vi "PickAndDestroy.vi"(0 "ImageIn":T1, 4 "Threshold":dbl=20.0 format="%.2f", 5 "Image":u32[][](array[numeric]), 6 "Image Settings":T4 {"2nd Axis" items=["x", "y", "z"]; "1st Axis" items=["x", "y", "z"]; "Time Resolution\n(ms/pixel)" format="%.2f"; "Image Resolution (nm/pixel)"."z" format="%.2f"; "Image Resolution (nm/pixel)"."y" format="%.2f"; "Image Resolution (nm/pixel)"."x" format="%.2f"; "Image Size (µm)"."z" format="%.2f"; "Image Size (µm)"."y" format="%.2f"; "Image Size (µm)"."x" format="%.2f"; "End Position (µm)"."z" format="%.2f"; "End Position (µm)"."y" format="%.2f"; "End Position (µm)"."x" format="%.2f"; "Start Position (µm)"."z" format="%.2f"; "Start Position (µm)"."y" format="%.2f"; "Start Position (µm)"."x" format="%.2f"}) -> ()   [LabVIEW 2009]
uses:
  ImageSettings.ctt
  <vilib>/vision/Image Controls.llb/IMAQ Image.ctl
  AO Update Channel (scaled value).vi
  <vilib>/ptbypt/NI_PtbyPt.lvlib
panel:
  out "spots left":i32
  out "Boolean":bool
  out "sum":i32
  in  "AutoFocus Z":bool
  in  "Delay Time (s)":dbl=120.0
  out "autofocus stub":i32[](array[numeric])
  out "Debug Image Ints":T1(plugin-control)
  out "Intensity for ft debug color/rotated by some angle":dbl[][](graph)
  out "Intensity fit gausian for SM":dbl[][](graph)
  in  "radius":i32
  out "Focuswidth/px":dbl
  in  "Treshold":dbl
  out "NrOfSpots":i32
  in  "Find Molecules":bool
  in  "Automate Mesaurement":bool
  in  "Focuswidth nm":dbl
  in  "AFM mode":bool
  in  "gauss fit":bool
  in  "channel":i32
  in  "initialize":bool
  out "Histogram Graph":T2(graph)
  in  ".sm file format":bool
  in  "manual positioning":cluster{"x":dbl, "y":dbl, "z":dbl}
  in  "Laser 4":bool
  out "used":bool
  in  "Ramp Setup":bool
  in  "% duration Laser1":u8=50 min=1 max=99
  in  "% puls-duration":dbl=100.0
  in  "Laser 3":bool
  in  "Laser 2":bool
  in  "Laser 1":bool
  in  "AOTF Setup":bool
  in  "AOTF":u16(ring)=1 items=["None", "Laser 1", "Laser 2", "Laser 1 + 2", "Laser 3", "Laser 1 + 3", "Laser 2 + 3", "Laser 1+2+3", "Laser 1+2+3+4", "Laser 2+3+4"]
  out "Pickcoord. (pixel)":cluster{dbl, dbl, dbl}
  in  "offset (pixel)":cluster{dbl, dbl, dbl}
  out "coordinates (pixel)":cluster{dbl, dbl, dbl}
  out "Actual Spot No.":u32
  in  "Store Pick Image":bool
  in  "Next":bool caption="Run"
  in  "Show MCS":bool=TRUE
  in  "Pick Settings":T3={"Automatic"=FALSE, "Threshold"=20.0, "radius"=0} {"Threshold" format="%.2f"}
  in  "Run":bool
  in  "Destination:":path
  in  "Store Data":bool caption="Store Data:"
  in  "Stage Setup":bool
  in  "SPC Setup":bool
  in  "EOM Setup":bool
  in  "EOM":u16(ring) items=["None", "Trace", "Retrace", "All"]
  out "Counts":cluster{"Total":u32, "Gap":u32, "Invalid":u32}
  out "MCS":i32[][](graph)
  in  "Exit":bool
  # "+"
  # "="
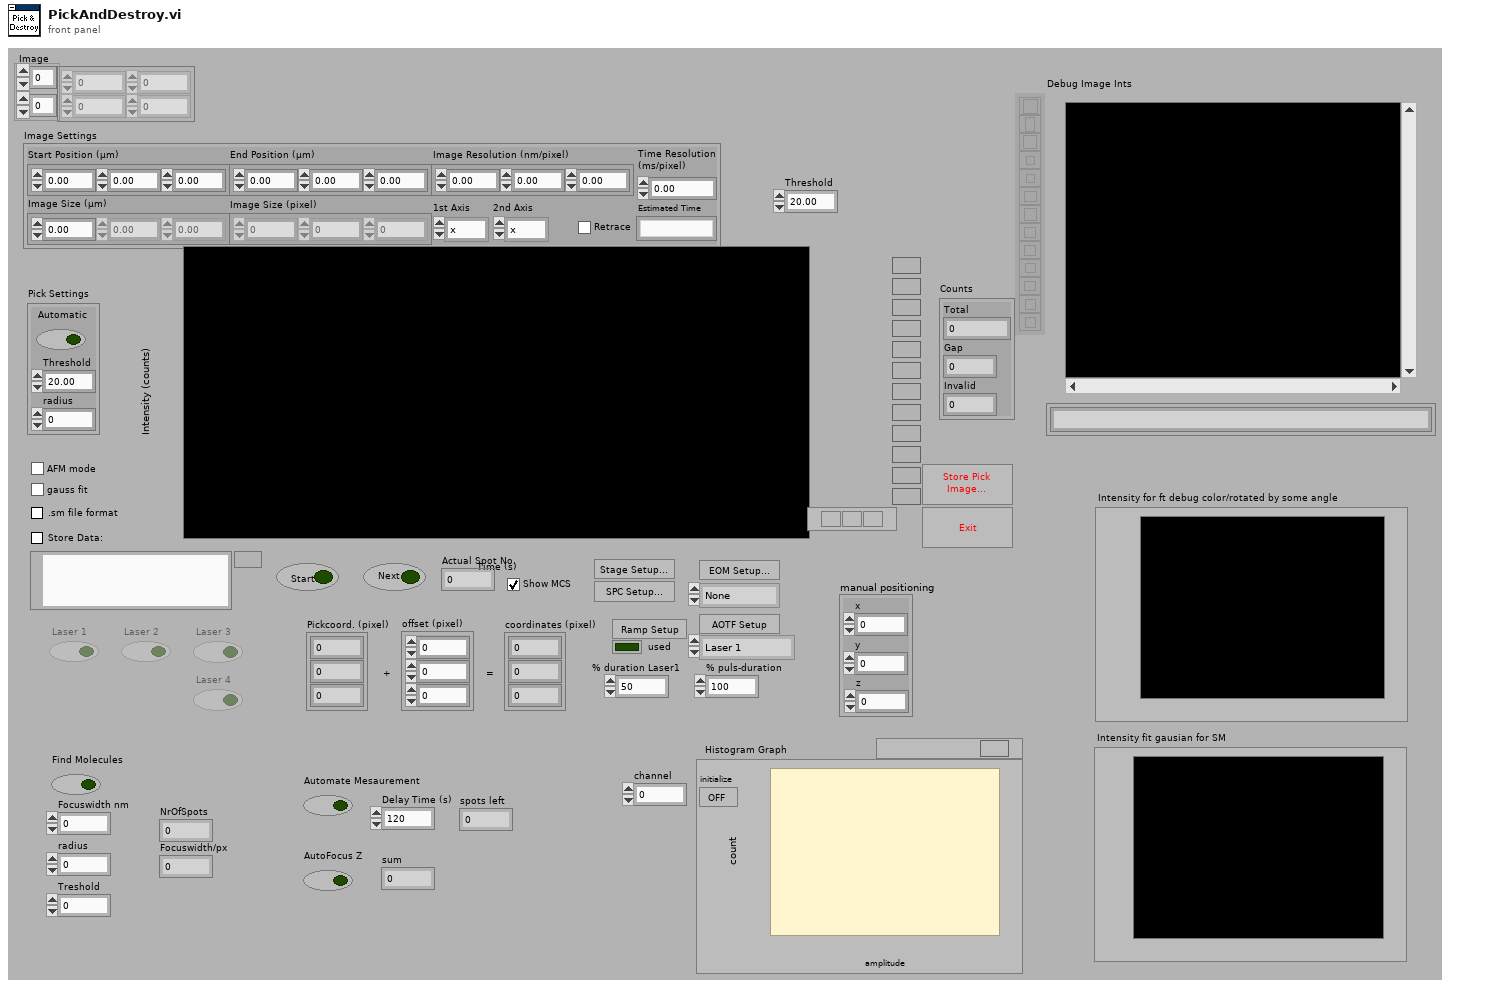
[diagram p1: front panel]
types:
  T1 = typedef "IMAQ Image.ctl" = refnum<image>
  T2 = cluster{"X Values":dbl[], "Histogram: h(x)":i32[]}
  T3 = cluster{"Automatic":bool, "Threshold":dbl, "radius":i32}
  T4 = typedef "ImageSettings.ctt" = cluster{"Start Position (µm)":cluster{"x":dbl, "y":dbl, "z":dbl}, "End Position (µm)":cluster{"x":dbl, "y":dbl, "z":dbl}, "Image Resolution (nm/pixel)":cluster{"x":dbl, "y":dbl, "z":dbl}, "Image Size (µm)":cluster{"x":dbl, "y":dbl, "z":dbl}, "Image Size (pixel)":cluster{"x":u32, "y":u32, "z":u32}, "Time Resolution\n(ms/pixel)":dbl, "1st Axis":u16, "2nd Axis":u16, "Retrace":bool, "Estimated Time":string}
  T5 = enum16{"Get Type", "Set Type", "GetStageInit", "GetWriteStageSetting", "GetInitializeStageOutput", "GetSetAxisPosition", "GetSetPos", "GetSetupStage", "HaltStageOutput"}
  T6 = typedef "FIFOSettings.ctt" = cluster{"Measurement":cluster{"Binning (ms)":sgl, "External Trigger Condition":u16, "Stop Condition:":u16, "Stop Count":dbl, "Buffer Size (Photons)":u32, "No of Channels":u16, "Ext Latch Delay":i16}, "ADC":cluster{"Binning (HH)":i16, "Dither Range":i16, "Count Increment":i16, "Mode":u16}, "SYNC":cluster{"SYNC ZC Level (mV)":sgl, "SYNC Freq Divider":u16, "SYNC Holdoff (ps)":sgl, "SYNC Threshold (mV)":sgl}, "TAC":cluster{"TAC Range (ns)":sgl, "TAC Gain":i16, "TAC Offset (%)":sgl, "TAC Limit Low (%)":sgl, "TAC Limit High (%)":sgl}, "Ch 2":cluster{"Ch2 ZC Level (mV)":sgl, "Ch2 Holdoff (ps)":sgl, "Ch2 Threshold (mV)":sgl}, "Ch 3":cluster{"Ch3 ZC Level (mV)":sgl, "Ch3 Holdoff (ps)":sgl, "Ch3 Threshold (mV)":sgl}, "Ch 4":cluster{"Ch4 ZC Level (mV)":sgl, "Ch4 Holdoff (ps)":sgl, "Ch4 Threshold (mV)":sgl}, "Ch1":cluster{"Ch1 ZC Level (mV)":sgl, "Ch1 Holdoff (ps)":sgl, "Ch1 Threshold (mV)":sgl}}
  T7 = typedef "PickImage.ctl" = cluster{"Rawdata":T1, "Mask":T1, "Display":T1, "Coefficients (2D)":sgl[][], "Destroy Index":u32}
  T8 = cluster{"Binning (ms)":sgl, "External Trigger Condition":u16, "Stop Condition:":u16, "Stop Count":dbl, "Buffer Size (Photons)":u32, "No of Channels":u16, "Ext Latch Delay":i16}
  T9 = cluster{"router channels":u8[], "macro times(50ns steps)":u32[], "micro times":u16[], "invalid times":u32[], "gap times":u32[]}
  T10 = cluster{"Start Position (µm)":cluster{"x":dbl, "y":dbl, "z":dbl}, "End Position (µm)":cluster{"x":dbl, "y":dbl, "z":dbl}, "Image Resolution (nm/pixel)":cluster{"x":dbl, "y":dbl, "z":dbl}, "Image Size (µm)":cluster{"x":dbl, "y":dbl, "z":dbl}, "Image Size (pixel)":cluster{"x":u32, "y":u32, "z":u32}, "Time Resolution\n(ms/pixel)":dbl, "1st Axis":u16, "2nd Axis":u16, "Retrace":bool, "Estimated Time":string}
  T11 = typedef "StageType.ctt" = enum16{"PI 725 USB", "PI 725 TCP/IP", "PI analogue step"}
  T12 = cluster{"used":bool, "steps":u16, "start (V)":dbl, "stop (V)":dbl, "periode (s)":dbl, "manual":dbl[][]}
  T13 = typedef "DAQLinescanVisualization.ctt" = cluster{"Threshold":u32, "Trace Window #":u32, "IMAQ Trace":T1, "Retrace Window #":u32, "IMAQ Retrace":T1}
  T14 = typedef "AOTFSettings.ctt" = cluster{"Laser 1 Output Channel":tag, "AOTF  1 Output Voltage":dbl, "Laser 2 Output Channel":tag, "AOTF  2 Output Voltage":dbl, "Laser 3 Output Channel":tag, "AOTF  3 Output Voltage":dbl, "Pixel per Cycle":u16, "Time per Cycle  / ms":dbl, "Laser 4 Output Channel":tag, "AOTF  4 Output Voltage":dbl, "Laser 5 Output Channel":tag, "AOTF 5 Output Voltage ":dbl, "Laser 6 Output Channel":tag, "AOTF  6 Output Voltage ":dbl, "Laser 7 Output Channel":tag, "AOTF 7 Output Voltage ":dbl, "Laser 8 Output Channel":tag, "AOTF  8 Output Voltage ":dbl, "AOTF  1 Frequency":dbl, "AOTF  2 Frequency":dbl, "AOTF  3  Frequency":dbl, "AOTF  4 Frequency":dbl, "AOTF 5 Frequency":dbl, "AOTF  6 Frequency":dbl, "AOTF 7  Frequency":dbl, "AOTF  8 Frequency":dbl, "AOTF  1 Amplitude":dbl, "AOTF  2 Amplitude":dbl, "AOTF  3  Amplitude":dbl, "AOTF  4 Amplitude":dbl, "AOTF 5 Amplitude":dbl, "AOTF  6 Amplitude":dbl, "AOTF 7 Amplitude  ":dbl, "AOTF  8 Amplitude":dbl}
  T15 = typedef "AnalogSettings.ctt" = cluster{"PCI 671x Device Number":u32, "Samples per Unit":u32}
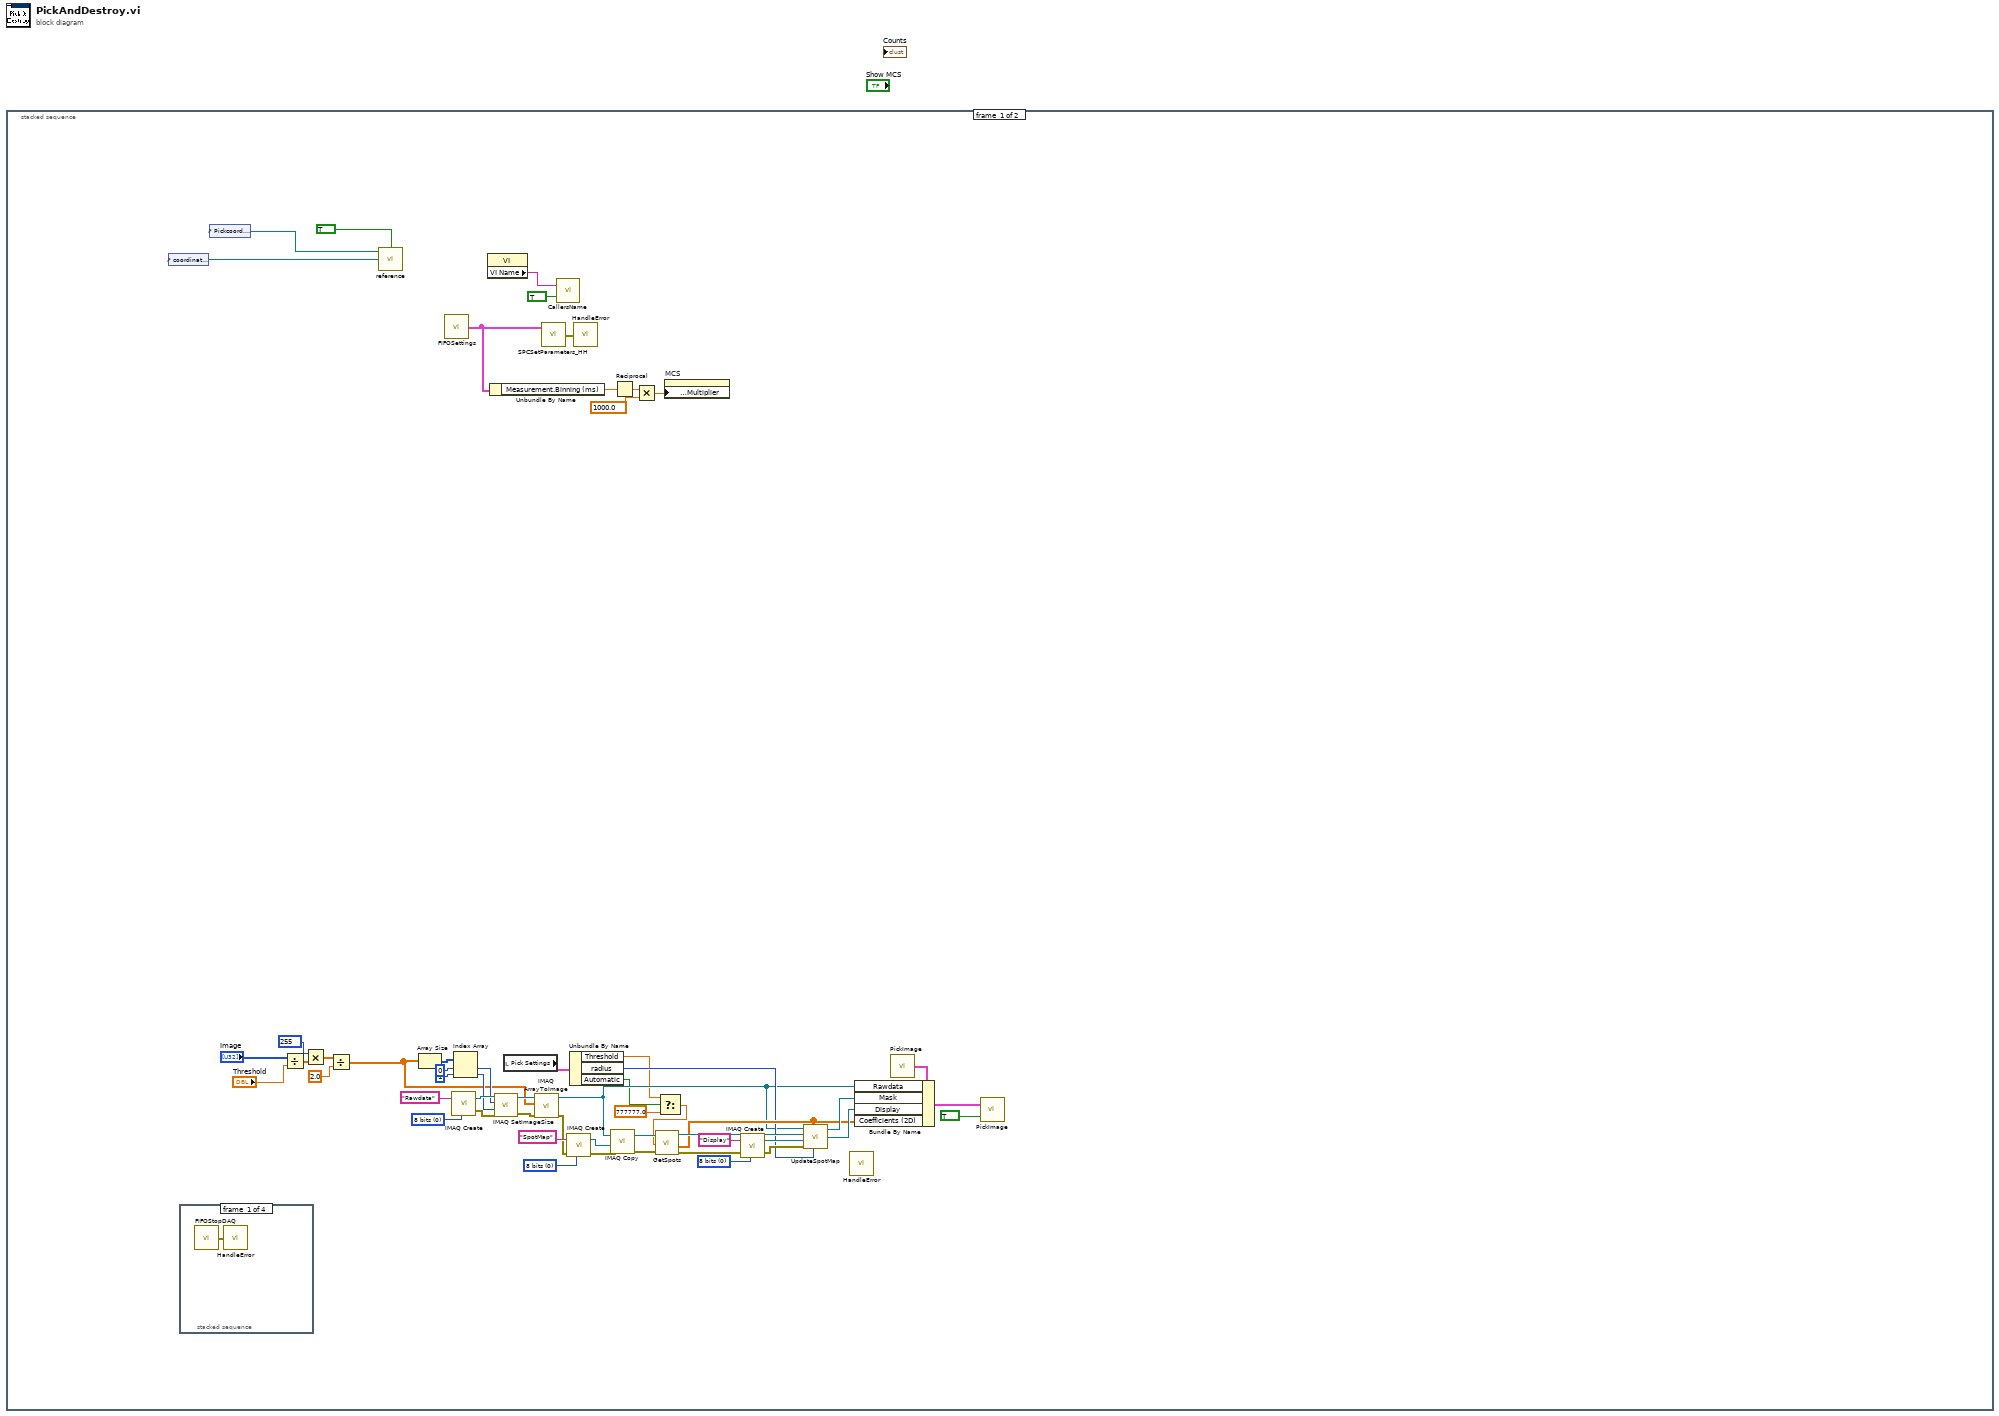
[diagram p0: block diagram]
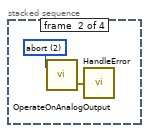
[diagram p2: hidden frame]
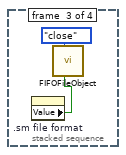
[diagram p3: hidden frame]
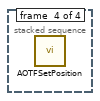
[diagram p4: hidden frame]
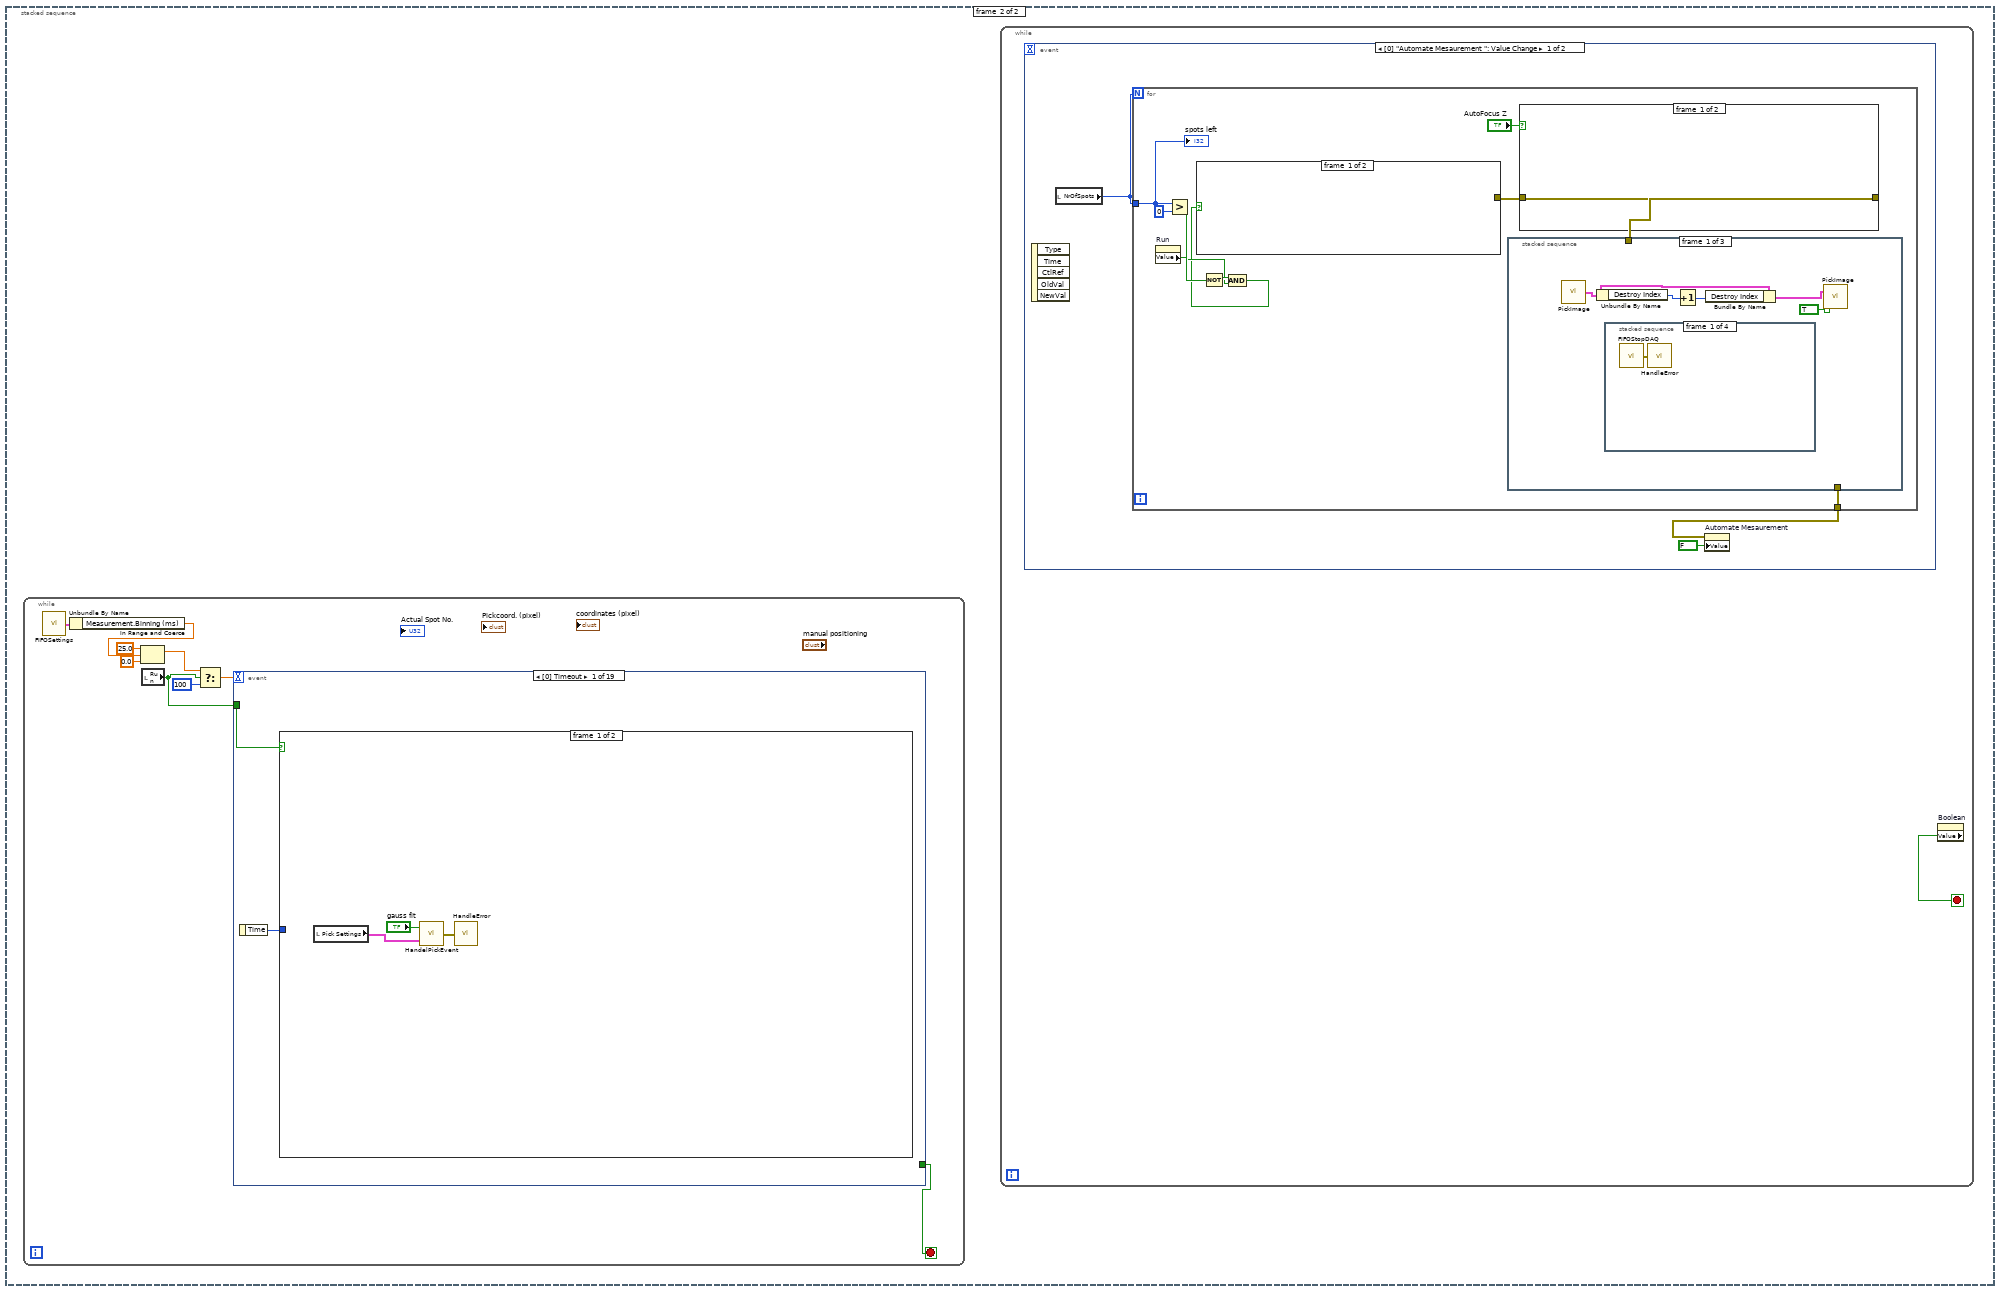
[diagram p5: hidden frame]
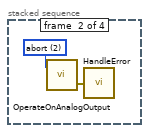
[diagram p6: hidden frame]
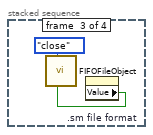
[diagram p7: hidden frame]
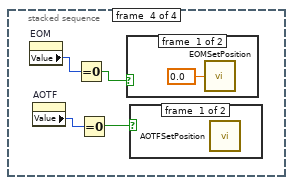
[diagram p8: hidden frame]
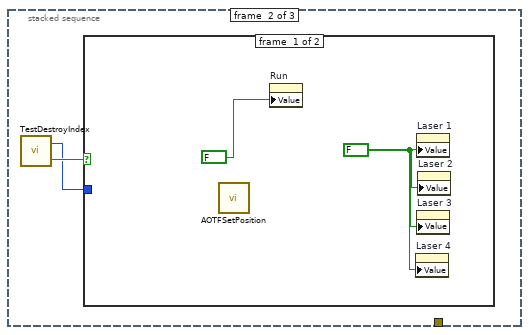
[diagram p11: hidden frame]
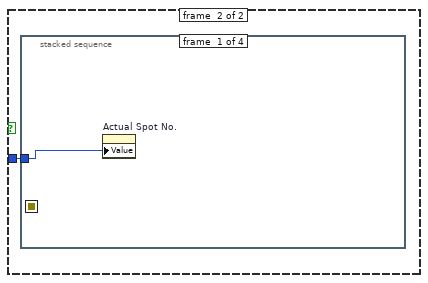
[diagram p12: hidden frame]
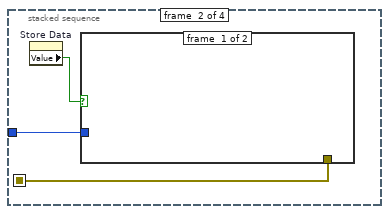
[diagram p13: hidden frame]
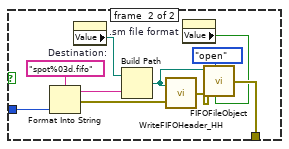
[diagram p14: hidden frame]
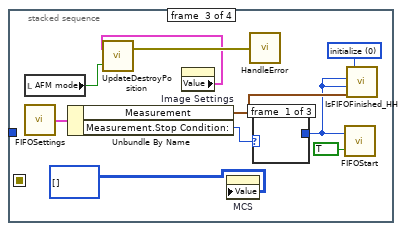
[diagram p15: hidden frame]
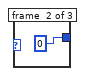
[diagram p16: hidden frame]
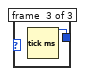
[diagram p17: hidden frame]
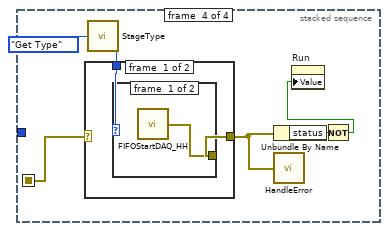
[diagram p18: hidden frame]
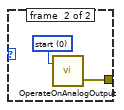
[diagram p19: hidden frame]
diagram:
  n1 = stacked-sequence {
    frame #0 {
      w39 = u32 0 items=["8 bits", "16 bits", "Float", "Complex", "RGB", "HSL"] ("Image Type")
      w44 = u32 0 items=["8 bits", "16 bits", "Float", "Complex", "RGB", "HSL"] ("Image Type")
      w54 = u32 0 items=["8 bits", "16 bits", "Float", "Complex", "RGB", "HSL"] ("Image Type")
      n2 = control-ref of="coordinates (pixel)"() -> (w16:refnum<vi>)
      n3 = stacked-sequence {
        frame #0 {
          n4 = call "FIFOStopDAQ.vi"() -> ("error out"=w56:errorcluster)
          n5 = call "HandleError.vi"("error in (no error)"=w56) -> ()
        }
        frame #1 {
          w58 = u16 2 items=["start", "state", "abort"] ("operation")
          n6 = call "OperateOnAnalogOutput.vi"("operation"=w58) -> ("error out"=w57:errorcluster)  [unwired: 1 in, 1 out]
          n7 = call "HandleError.vi"("error in (no error)"=w57) -> ()
        }
        frame #2 {
          n8 = property on=".sm file format" class="Bool (strict)"() -> ("Value"=w59:bool)  [unwired: 2 in, 2 out]
          n9 = call "FIFOFileObject.vi"(".sm file format"=w59, "function (open:0)"=enum16{"open", "write", "close"}."close") -> ()  [unwired: 4 in, 1 out]
        }
        frame #3 {
          n10 = call "AOTFSetPosition.vi"() -> ()  [unwired: 2 in]
        }
      }
      n11 = control-ref of="Pickcoord. (pixel)"() -> (w17:refnum<vi>)
      n12 = Divide(x="Image", y="Threshold") -> (x/y=w22:dbl[][])
      n13 = Multiply(x=u8 255, y=w22) -> (x*y=w7:dbl[][])
      n14 = Divide(x=w7, y=2.0) -> (x/y=w5:dbl[][])
      n15 = call "reference.vi"("set?"=TRUE, "coordinates (pixel)"=w16, "Pickcoord. (pixel)"=w17) -> ()  [unwired: 1 in, 2 out]
      n16 = Array Size(array=w5) -> (size(s)=w53:i32[])
      n17 = call "FIFOSettings.vi"() -> ("FIFO Settings(out)"=w14:T6)  [unwired: 2 in]
      n18 = call "IMAQ Create"("Image Name"="Rawdata", "Image Type"=w54) -> ("New Image"=w50:T1, "error out"=w49:errorcluster)  [unwired: 3 in]
      n19 = Index Array(array=w53, index #1=0 ("index"), index #2=1 ("index")) -> (element #1=w8:i32, element #2=w38:i32)
      n20 = property class="VI"() -> ("VI Name"=w18:string)  [unwired: 2 in, 2 out]
      n21 = Unbundle By Name(w14) -> ("Measurement.Binning (ms)"=w13:sgl)
      n22 = call "IMAQ SetImageSize"("error in (no error)"=w49, "Y Resolution"=w38, "X Resolution"=w8, "Image"=w50) -> ("error out"=w47:errorcluster, "Image Out"=w48:T1)  [unwired: 1 in]
      n23 = local read "Pick Settings"() -> (w26:T3)
      n24 = call "IMAQ ArrayToImage"("error in (no error)"=w47, "Image Pixels (U8)"=w5, "Image"=w48) -> ("error out"=w41:errorcluster, "Image Out"=w9:T1)  [unwired: 7 in]
      n25 = call "SPCSetParameters_HH.vi"("FIFO Settings"=w14) -> ("error (out)"=w24:errorcluster)  [unwired: 2 in]
      n26 = call "CallersName.vi"("Get/Set"=TRUE ("s"), "Callers Name"=w18) -> ()  [unwired: 1 out]
      n27 = call "IMAQ Create"("Image Name"="SpotMap", "Image Type"=w44, "error in (no error)"=w41) -> ("New Image"=w37:T1, "error out"=w36:errorcluster)  [unwired: 2 in]
      n28 = Unbundle By Name(w26) -> ("Threshold"=w4:dbl, "radius"=w25:i32, "Automatic"=w3:bool)
      n29 = call "HandleError.vi"("error in (no error)"=w24) -> ()
      n30 = call "IMAQ Copy"("error in (no error)"=w36, "Image Dst"=w37, "Image Src"=w9) -> ("error out"=w34:errorcluster, "Image Dst Out"=w35:T1)  [unwired: 3 in]
      n31 = Reciprocal(x=w13) -> (1/x=w12:sgl)
      n32 = Multiply(x=w12, y=sgl 1000.0) -> (x*y=w11:sgl)
      n33 = Select(t=w4, s=w3, f=777777.0) -> (s? t:f=w1:dbl)
      n34 = call "GetSpots.vi"("New Image"=w35, "Threshold"=w1, "error in (no error)"=w34) -> ("Image Dst Out"=w30:T1, "Coefficients (2D)"=w27:sgl[][], "error out"=w33:errorcluster)  [unwired: 2 out]
      n35 = property on="MCS" class="WFChart (strict)"("X Scale.Offset and Multiplier:Multiplier"=w11) -> ()  [unwired: 2 in, 2 out]
      n36 = call "IMAQ Create"("Image Name"="Display", "Image Type"=w39, "error in (no error)"=w33) -> ("New Image"=w31:T1, "error out"=w32:errorcluster)  [unwired: 2 in]
      n37 = call "UpdateSpotMap.vi"("Rawdata"=w9, "Coefficients"=w27, "Mask (input)"=w30, "Display Input"=w31, "radius"=w25, "error in (no error)"=w32) -> ("Mask (output)"=w29:T1, "Display (output"=w28:T1)  [unwired: 1 out]
      n38 = call "HandleError.vi"() -> ()  [unwired: 1 in]
      n39 = call "PickImage.vi"() -> ("Image (output)"=w46:T7)  [unwired: 2 in]
      n40 = Bundle By Name(cluster=w46, "Rawdata"=w9, "Mask"=w29, "Display"=w28, "Coefficients (2D)"=w27) -> (w42:T7)
      n41 = call "PickImage.vi"("Get/Set"=TRUE, "Images (input)"=w42) -> ()  [unwired: 1 out]
    }
    frame #1 {
      n42 = while {
        stop <- w154 stop-if-true
        n43 = call "FIFOSettings.vi"() -> ("FIFO Settings(out)"=w150:T6)  [unwired: 2 in]
        n44 = Unbundle By Name(w150) -> ("Measurement.Binning (ms)"=w147:sgl)
        n45 = In Range and Coerce(upper limit=25.0, x=w147, lower limit=0.0) -> (coerced(x)=w146:dbl)  [unwired: 1 out]
        n46 = local read "Run"() -> (w151:bool)
        n47 = Select(t=w146, s=w151, f=100) -> (s? t:f=w152:dbl)
        n48 = event shown="[0] Timeout" {
          selector: _ -> [_ _ _ _ _ _ _ _ _ _ _ _ _ _ _ _ _ _ _]
          dyn-events: _ -> [_ _ _ _ _ _ _ _ _ _ _ _ _ _ _ _ _ _ _]
          timeout: w152 -> [_ _ _ _ _ _ _ _ _ _ _ _ _ _ _ _ _ _ _]
          tunnel: [_ _ _ _ _ _ _ _ _ _ _ _ _ _ _ _ _ _ w534] -> w154
          tunnel: w151 -> [w156 _ _ _ _ _ _ _ _ _ _ _ _ _ _ _ _ _ _]
          event #0 {
            n49 = event-data() -> ("Time"=w155:u32)  [unwired: 1 in]
            n50 = case shown="True" w156 {
              tunnel: w155 -> [_ w160]
              frame #0 {
                n51 = local read "Pick Settings"() -> (w159:T3)
                n52 = call "HandelPickEvent.vi"("Pick Settings"=w159, "gauss fit"="gauss fit") -> ("error out"=w158:errorcluster)
                n53 = call "HandleError.vi"("error in (no error)"=w158) -> ()
              }
              frame #1 {
                n54 = call "IsSPCArmed_HH.vi"() -> ("Boolean"=w161:bool)  [unwired: 1 in]
                n55 = case shown="True" w161 {
                  tunnel: w160 -> [w164 w206]
                  frame #0 {
                    n56 = call "TestDestroyIndex.vi"() -> ("Boolean"=w163:bool, "Destroy Index"=w162:u32)
                    n57 = case shown="True" w163 {
                      selector: w163 -> [w165 _]
                      tunnel: w164 -> [_ _]
                      tunnel: w162 -> [_ w171]
                      frame #0 {
                        n58 = property on="Run" class="Boolean (strict)"("Value"=w165) -> ()  [unwired: 2 in, 2 out]
                        n59 = stacked-sequence {
                          frame #0 {
                            n60 = call "FIFOStopDAQ.vi"() -> ("error out"=w166:errorcluster)
                            n61 = call "HandleError.vi"("error in (no error)"=w166) -> ()
                          }
                          frame #1 {
                            w168 = u16 2 items=["start", "state", "abort"] ("operation")
                            n62 = call "OperateOnAnalogOutput.vi"("operation"=w168) -> ("error out"=w167:errorcluster)  [unwired: 1 in, 1 out]
                            n63 = call "HandleError.vi"("error in (no error)"=w167) -> ()
                          }
                          frame #2 {
                            n64 = property on=".sm file format" class="Bool (strict)"() -> ("Value"=w169:bool)  [unwired: 2 in, 2 out]
                            n65 = call "FIFOFileObject.vi"(".sm file format"=w169, "function (open:0)"=enum16{"open", "write", "close"}."close") -> ()  [unwired: 4 in, 1 out]
                          }
                          frame #3 {
                            n66 = call "AOTFSetPosition.vi"() -> ()  [unwired: 2 in]
                            n67 = call "EOMSetPosition.vi"() -> ()  [unwired: 1 in]
                          }
                        }
                      }
                      frame #1 {
                        n68 = stacked-sequence {
                          seq-local: [w173 _ _] -> [_ _ w200]
                          tunnel: w171 -> [w172 _ _]
                          frame #0 {
                            n69 = case shown="True" "Store Data" {
                              tunnel: [_ w182] -> w173
                              tunnel: w172 -> [_ w177]
                              frame #0 {
                              }
                              frame #1 {
                                n70 = Format Into String(format string="spot%03d.fifo", w177) -> (resulting string=w179:string, error out=w178:errorcluster)  [unwired: 2 in]
                                n71 = Build Path(base path="Destination:", name or relative path=w179) -> (appended path=w176:path)
                                n72 = property on=".sm file format" class="Bool (strict)"() -> ("Value"=w175:bool)  [unwired: 2 in, 2 out]
                                n73 = call "WriteFIFOHeader_HH.vi"("error in"=w178, "Destination:"=w176) -> ("error out"=w183:errorcluster)
                                n74 = call "FIFOFileObject.vi"(".sm file format"=w175, "function (open:0)"=enum16{"open", "write", "close"}."open", "error in (no error)"=w183, "Destination:"=w176) -> ("error out"=w182:errorcluster)  [unwired: 2 in]
                              }
                            }
                          }
                          frame #1 {
                            w190 = u16 0 items=["initialize", "test limit"] ("operation")
                            n75 = call "FIFOSettings.vi"() -> ("FIFO Settings(out)"=w191:T6)  [unwired: 2 in]
                            n76 = local read "AFM mode"() -> (w185:bool)
                            n77 = Unbundle By Name(w191) -> ("Measurement"=w189:T8, "Measurement.Stop Condition:"=w192:u16)
                            n78 = call "UpdateDestroyPosition.vi"("AFM Mode"=w185, "Image Settings"="Image Settings") -> ("error out"=w186:errorcluster)  [unwired: 1 in]
                            n79 = property on="MCS" class="WFChart (strict)"("History Data"=u32[][] []) -> ()  [unwired: 2 in, 2 out]
                            n80 = call "HandleError.vi"("error in (no error)"=w186) -> ()
                            n81 = case shown="2" w192 {
                              tunnel: [_ u32 0 ("Start (input)") w196] -> w187
                              frame #0 {
                              }
                              frame #1 {
                              }
                              frame #2 {
                                n82 = Tick Count (ms)() -> (millisecond timer value=w196:u32)
                              }
                            }
                            n83 = call "FIFOStart.vi"("Set/Get"=TRUE, "Start (input)"=w187) -> ()  [unwired: 1 out]
                            n84 = call "IsFIFOFinished_HH.vi"("Measurement"=w189, "Time"=w187, "Counts"=w187, "operation"=w190) -> ()  [unwired: 1 out]
                          }
                          frame #2 {
                            n85 = case shown="No Error" w200 {
                              selector: w200 -> [_ w203]
                              tunnel: [w201 w203] -> w197
                              frame #0 {
                                w202 = u16 0 items=["start", "state", "abort"] ("operation")
                                n86 = call "OperateOnAnalogOutput.vi"("operation"=w202) -> ("error out"=w201:errorcluster)  [unwired: 1 in, 1 out]
                              }
                              frame #1 {
                              }
                            }
                            n87 = Unbundle By Name(w197) -> ("status"=w199:bool)
                            n88 = call "HandleError.vi"("error in (no error)"=w197) -> ()
                            n89 = Not(x=w199) -> (.not. x?=w198:bool)
                            n90 = property on="Run" class="Boolean (strict)"("Value"=w198) -> ()  [unwired: 2 in, 2 out]
                          }
                        }
                      }
                    }
                  }
                  frame #1 {
                    w216 = u16 1 items=["initialize", "test limit"] ("operation")
                    # "ADC module"
                    n91 = case shown="True" TRUE ("Case Constant\n(See Context Help)") {
                      tunnel: [_ w229] -> w205
                      frame #0 {
                      }
                      frame #1 {
                        w228 = u16 1 items=["init", "run"] ("mode")
                        n92 = property on=".sm file format" class="Bool (strict)"() -> ("Value"=w234:bool)  [unwired: 2 in, 2 out]
                        n93 = property on="Store Data" class="Boolean (strict)"() -> ("Value"=w235:bool)  [unwired: 2 in, 2 out]
                        n94 = call "SPCReadFIFO_HH.vi"() -> ("count"=w229:i32, "error out"=w236:errorcluster, "buffer"=w230:u32[])  [unwired: 2 in]
                        n95 = case shown="False" w235 {
                          tunnel: [w245 w251] -> w237
                          tunnel: w236 -> [w245 w250]
                          tunnel: w230 -> [_ w248]
                          tunnel: w229 -> [_ w247]
                          tunnel: w234 -> [_ w246]
                          frame #0 {
                          }
                          frame #1 {
                            n96 = call "FIFOFileObject.vi"(".sm file format"=w246, "function (open:0)"=enum16{"open", "write", "close"}."write", "error in (no error)"=w250, "count"=w247, "buffer"=w248) -> ("error out"=w251:errorcluster)  [unwired: 1 in]
                          }
                        }
                        n97 = Array Subset(array=w230, index=0, length=w229) -> (w232:u32[])
                        n98 = call "ParseFIFO_HH.vi"("RawData"=w232) -> ("RawData Out"=w231:T9)  [unwired: 1 in]
                        n99 = call "HandleError.vi"("error in (no error)"=w237) -> ()
                        n100 = call "_updateOnlineDisplay_LV.vi"("show lifetime"=FALSE, "Raw Data"=w231, "mode"=w228) -> ("Timetraces"=w226:i32[][])  [unwired: 1 in, 1 out]
                        "MCS" <- w226
                        n101 = Index Array(array=w226, index (row)="channel") -> (element=w224:i32[])  [unwired: 1 in]
                        "autofocus stub" <- w224
                        n102 = for {
                          tunnel: w224 -> [w240] mode=indexing
                          tunnel: 1000 ("sample length") -> [w243]
                          tunnel: "initialize" -> [w242]
                          n103 = call <vilib>:"Histogram PtByPt.vi"("initialize"=w242, "sample length"=w243, "intervals"=10, "x"=w240) -> ("Histogram Graph"=→"Histogram Graph":T2)  [unwired: 4 in, 3 out]
                          n104 = Equal To 0?(x=w240) -> (x = 0?=w239:bool)
                          n105 = case shown="False" w239 {
                            tunnel: w239 -> [_ w244]
                            tunnel: [_ w244] -> _
                            frame #0 {
                            }
                            frame #1 {
                            }
                          }
                        }
                      }
                    }
                    n106 = call "FIFOSettings.vi"() -> ("FIFO Settings(out)"=w214:T6)  [unwired: 2 in]
                    n107 = Unbundle By Name(w214) -> ("ADC.Dither Range"=w208:i16)
                    n108 = Equal To 0?(x=w208) -> (x = 0?=w209:bool)
                    n109 = Select(t=2, s=w209, f=3) -> (s? t:f=w212:i32)
                    n110 = Divide(x=w205, y=w212) -> (x/y=w213:dbl)
                    n111 = To Unsigned Long Integer(number=w213) -> (unsigned 32bit integer=w215:u32)
                    n112 = call "IsFIFOFinished_HH.vi"("Time"=w206, "Counts"=w215, "operation"=w216) -> ("Boolean"=w207:bool)  [unwired: 1 in]
                    n113 = case shown="False" w207 {
                      frame #0 {
                      }
                      frame #1 {
                        n114 = stacked-sequence {
                          frame #0 {
                            n115 = call "FIFOStopDAQ.vi"() -> ("error out"=w217:errorcluster)
                            n116 = call "HandleError.vi"("error in (no error)"=w217) -> ()
                          }
                          frame #1 {
                            w219 = u16 2 items=["start", "state", "abort"] ("operation")
                            n117 = call "OperateOnAnalogOutput.vi"("operation"=w219) -> ("error out"=w218:errorcluster)  [unwired: 1 in, 1 out]
                            n118 = call "HandleError.vi"("error in (no error)"=w218) -> ()
                          }
                          frame #2 {
                            n119 = property on=".sm file format" class="Bool (strict)"() -> ("Value"=w220:bool)  [unwired: 2 in, 2 out]
                            n120 = call "FIFOFileObject.vi"(".sm file format"=w220, "function (open:0)"=enum16{"open", "write", "close"}."close") -> ()  [unwired: 4 in, 1 out]
                          }
                        }
                      }
                    }
                  }
                }
              }
            }
          }
          event #1 {
            n121 = event-data() -> ()  [unwired: 1 in, 5 out]
            n122 = stacked-sequence {
              tunnel: w252 -> [_ _]
              frame #0 {
                n123 = call "PickImage.vi"() -> ("Image (output)"=w261:T7)  [unwired: 2 in]
                n124 = Unbundle By Name(w261) -> ("Destroy Index"=w259:u32)
                n125 = stacked-sequence {
                  frame #0 {
                    n126 = call "FIFOStopDAQ.vi"() -> ("error out"=w263:errorcluster)
                    n127 = call "HandleError.vi"("error in (no error)"=w263) -> ()
                  }
                  frame #1 {
                    w265 = u16 2 items=["start", "state", "abort"] ("operation")
                    n128 = call "OperateOnAnalogOutput.vi"("operation"=w265) -> ("error out"=w264:errorcluster)  [unwired: 1 in, 1 out]
                    n129 = call "HandleError.vi"("error in (no error)"=w264) -> ()
                  }
                  frame #2 {
                    n130 = property on=".sm file format" class="Bool (strict)"() -> ("Value"=w266:bool)  [unwired: 2 in, 2 out]
                    n131 = call "FIFOFileObject.vi"(".sm file format"=w266, "function (open:0)"=enum16{"open", "write", "close"}."close") -> ()  [unwired: 4 in, 1 out]
                  }
                  frame #3 {
                    n132 = property on="EOM" class="Ring (strict)"() -> ("Value"=w270:u16)  [unwired: 2 in, 2 out]
                    n133 = property on="AOTF" class="Ring (strict)"() -> ("Value"=w268:u16)  [unwired: 2 in, 2 out]
                    n134 = Equal To 0?(x=w270) -> (x = 0?=w271:bool)
                    n135 = Equal To 0?(x=w268) -> (x = 0?=w269:bool)
                    n136 = case shown="True" w271 {
                      frame #0 {
                        n137 = call "EOMSetPosition.vi"("value"=sgl 0.0) -> ()
                      }
                      frame #1 {
                      }
                    }
                    n138 = case shown="False" w269 {
                      frame #0 {
                        n139 = call "AOTFSetPosition.vi"() -> ()  [unwired: 2 in]
                      }
                      frame #1 {
                      }
                    }
                  }
                }
                n140 = Increment(x=w259) -> (x+1=w260:u32)
                n141 = Bundle By Name(cluster=w261, "Destroy Index"=w260) -> (w262:T7)
                n142 = call "PickImage.vi"("Get/Set"=TRUE, "Images (input)"=w262) -> ()  [unwired: 1 out]
              }
              frame #1 {
                n143 = call "TestDestroyIndex.vi"() -> ("Boolean"=w274:bool, "Destroy Index"=w273:u32)
                n144 = case shown="False" w274 {
                  tunnel: w273 -> [_ w277]
                  frame #0 {
                    w275 = FALSE ("Laser 1")
                    n145 = call "AOTFSetPosition.vi"() -> ()  [unwired: 2 in]
                    n146 = property on="Run" class="Bool (strict)"("Value"=FALSE ("Run")) -> ()  [unwired: 2 in, 2 out]
                    n147 = property on="Laser 1" class="Boolean (strict)"("Value"=w275) -> ()  [unwired: 2 in, 2 out]
                    n148 = property on="Laser 2" class="Boolean (strict)"("Value"=w275) -> ()  [unwired: 2 in, 2 out]
                    n149 = property on="Laser 3" class="Boolean (strict)"("Value"=w275) -> ()  [unwired: 2 in, 2 out]
                    n150 = property on="Laser 4" class="Boolesch (strikt)"("Value"=w275) -> ()  [unwired: 2 in, 2 out]
                  }
                  frame #1 {
                    n151 = stacked-sequence {
                      seq-local: [_ w281 _ _] -> [_ _ _ w309]
                      tunnel: w277 -> [w278 w279 _ _]
                      frame #0 {
                        n152 = property on="Actual Spot No." class="Digital (strict)"("Value"=w278) -> ()  [unwired: 2 in, 2 out]
                      }
                      frame #1 {
                        n153 = property on="Store Data" class="Boolean (strict)"() -> ("Value"=w280:bool)  [unwired: 2 in, 2 out]
                        n154 = case shown="False" w280 {
                          tunnel: [_ w289] -> w281
                          tunnel: w279 -> [_ w285]
                          frame #0 {
                          }
                          frame #1 {
                            n155 = property on="Destination:" class="Path"() -> ("Value"=w286:path)  [unwired: 2 in, 2 out]
                            n156 = Format Into String(format string="spot%03d.fifo", w285) -> (resulting string=w287:string, error out=w282:errorcluster)  [unwired: 2 in]
                            n157 = Build Path(base path=w286, name or relative path=w287) -> (appended path=w284:path)
                            n158 = property on=".sm file format" class="Bool (strict)"() -> ("Value"=w283:bool)  [unwired: 2 in, 2 out]
                            n159 = call "WriteFIFOHeader_HH.vi"("error in"=w282, "Destination:"=w284) -> ("error out"=w290:errorcluster)
                            n160 = call "FIFOFileObject.vi"(".sm file format"=w283, "function (open:0)"=enum16{"open", "write", "close"}."open", "error in (no error)"=w290, "Destination:"=w284) -> ("error out"=w289:errorcluster)  [unwired: 2 in]
                          }
                        }
                      }
                      frame #2 {
                        w298 = u16 0 items=["initialize", "test limit"] ("operation")
                        n161 = property on="Image Settings" class="Cluster (strict)"() -> ("Value"=w294:T10)  [unwired: 2 in, 2 out]
                        n162 = local read "AFM mode"() -> (w292:bool)
                        n163 = call "FIFOSettings.vi"() -> ("FIFO Settings(out)"=w299:T6)  [unwired: 2 in]
                        n164 = Unbundle By Name(w299) -> ("Measurement"=w297:T8, "Measurement.Stop Condition:"=w300:u16)
                        n165 = call "UpdateDestroyPosition.vi"("AFM Mode"=w292, "Image Settings"=w294) -> ("error out"=w293:errorcluster)  [unwired: 1 in]
                        n166 = property on="MCS" class="WFChart (strict)"("History Data"=u32[][] []) -> ()  [unwired: 2 in, 2 out]
                        n167 = call "HandleError.vi"("error in (no error)"=w293) -> ()
                        n168 = case shown="2" w300 {
                          tunnel: [_ u32 0 ("Start (input)") w303] -> w295
                          frame #0 {
                          }
                          frame #1 {
                          }
                          frame #2 {
                            n169 = Tick Count (ms)() -> (millisecond timer value=w303:u32)
                          }
                        }
                        n170 = call "FIFOStart.vi"("Set/Get"=TRUE, "Start (input)"=w295) -> ()  [unwired: 1 out]
                        n171 = call "IsFIFOFinished_HH.vi"("Measurement"=w297, "Time"=w295, "Counts"=w295, "operation"=w298) -> ()  [unwired: 1 out]
                      }
                      frame #3 {
                        n172 = call "StageType.vi"("Function"=T5."Get Type") -> ("Stage Type (output)"=w304:T11)  [unwired: 2 in, 2 out]
                        n173 = case shown="No Error" w309 {
                          selector: w309 -> [_ w315]
                          tunnel: [w311 w315] -> w306
                          tunnel: w304 -> [w310 _]
                          frame #0 {
                            n174 = case shown="\"PI 725 TCP/IP\", Default" w310 {
                              tunnel: [w312 w313] -> w311
                              frame #0 {
                                n175 = call "FIFOStartDAQ_HH.vi"() -> ("error out"=w312:errorcluster)  [unwired: 1 in]
                              }
                              frame #1 {
                                w314 = u16 0 items=["start", "state", "abort"] ("operation")
                                n176 = call "OperateOnAnalogOutput.vi"("operation"=w314) -> ("error out"=w313:errorcluster)  [unwired: 1 in, 1 out]
                              }
                            }
                          }
                          frame #1 {
                          }
                        }
                        n177 = Unbundle By Name(w306) -> ("status"=w308:bool)
                        n178 = call "HandleError.vi"("error in (no error)"=w306) -> ()
                        n179 = Not(x=w308) -> (.not. x?=w307:bool)
                        n180 = property on="Run" class="Bool (strict)"("Value"=w307) -> ()  [unwired: 2 in, 2 out]
                      }
                    }
                  }
                }
              }
            }
            n181 = flat-sequence {
              tunnel: "Next" -> [w256]
              tunnel: [w254] -> w252
              frame #0 {
                n182 = case shown="True" w256 {
                  frame #0 {
                  }
                  frame #1 {
                    n183 = Wait (ms)(milliseconds to wait=u32 500) -> ()  [unwired: 1 out]
                  }
                }
                n184 = property on="Next" class="Bool (strict)"("Value"=FALSE ("Next")) -> (error out=w254:errorcluster)  [unwired: 2 in, 1 out]
              }
            }
          }
          event #2 {
            n185 = event-data() -> ()  [unwired: 1 in, 5 out]
            n186 = call "PickImage.vi"() -> ("Image (output)"=w317:T7)  [unwired: 2 in]
            n187 = stacked-sequence {
              tunnel: w317 -> [_ w338 _]
              tunnel: "Pick Settings" -> [w319 _ w339]
              frame #0 {
                n188 = Bundle By Name(cluster=w319, "Automatic"=TRUE) -> (w320:T3)
                n189 = local write "Pick Settings"(w320) -> ()
              }
              frame #1 {
                n190 = local read "Pick Settings"() -> (w323:T3)
                n191 = Unbundle By Name(w338) -> ("Rawdata"=w331:T1, "Mask"=w332:T1, "Display"=w329:T1)
                n192 = Unbundle By Name(w323) -> ("Threshold"=w322:dbl, "radius"=w321:i32)
                n193 = call "IMAQ Copy"("Image Dst"=w332, "Image Src"=w331) -> ("error out"=w333:errorcluster, "Image Dst Out"=w334:T1)  [unwired: 4 in]
                n194 = call "GetSpots.vi"("New Image"=w334, "Threshold"=w322, "error in (no error)"=w333) -> ("Image Dst Out"=w330:T1, "Coefficients (2D)"=w324:sgl[][], "error out"=w328:errorcluster)  [unwired: 2 out]
                n195 = call "UpdateSpotMap.vi"("Rawdata"=w331, "Coefficients"=w324, "Mask (input)"=w330, "Display Input"=w329, "radius"=w321, "error in (no error)"=w328) -> ("Mask (output)"=w327:T1, "Display (output"=w326:T1, "error out"=w325:errorcluster)
                n196 = call "HandleError.vi"("error in (no error)"=w325) -> ()
                n197 = call "PickImage.vi"() -> ("Image (output)"=w337:T7)  [unwired: 2 in]
                n198 = Bundle By Name(cluster=w337, "Mask"=w327, "Display"=w326, "Coefficients (2D)"=w324) -> (w335:T7)
                n199 = call "PickImage.vi"("Get/Set"=TRUE, "Images (input)"=w335) -> ()  [unwired: 1 out]
              }
              frame #2 {
                n200 = Bundle By Name(cluster=w339, "Automatic"=FALSE) -> (w341:T3)
                n201 = local write "Pick Settings"(w341) -> ()
              }
            }
          }
          event #3 {
            n202 = event-data() -> ()  [unwired: 1 in, 5 out]
            n203 = call "PickImage.vi"() -> ("Image (output)"=w371:T7)  [unwired: 2 in]
            n204 = local read "Image Settings"() -> (w359:T4)
            n205 = Unbundle By Name(w359) -> ("Image Resolution (nm/pixel).x"=w356:dbl)
            n206 = Unbundle By Name(w371) -> ("Rawdata"=w364:T1, "Mask"=w363:T1, "Display"=w343:T1)
            "Debug Image Ints" <- w343
            n207 = call "IMAQ Copy"("Image Dst"=w363, "Image Src"=w364) -> ("error out"=w366:errorcluster, "Image Dst Out"=w344:T1)  [unwired: 4 in]
            n208 = Divide(x="Focuswidth nm", y=w356) -> (x/y=w352:dbl)
            "Focuswidth/px" <- w352
            n209 = call "SIMA.vi"("error in"=w366, "tsh"="Treshold", "focus"=w352, "In"="ImageIn") -> ("error out"=w365:errorcluster, "Out"=w345:T1, "Intensity fit gausian for SM"=→"Intensity fit gausian for SM":dbl[][], "Coefficiens"=w350:dbl[][], "Intensity for ft debug color"=→"Intensity for ft debug color/rotated by some angle":dbl[][])  [unwired: 3 in]
            n210 = Index Array(array=w350, index (row) #1=0 ("index"), index (row) #2=1 ("index (row)")) -> (element #1=w348:dbl[], element #2=w347:dbl[])  [unwired: 2 in]
            n211 = Array Size(array=w348) -> (size(s)=w349:i32)
            "NrOfSpots" <- w349
            n212 = call "PickImage.vi"() -> ("Image (output)"=w370:T7)  [unwired: 2 in]
            n213 = for {
              N: w349 -> [_]
              tunnel: w348 -> [w372] mode=indexing
              tunnel: w347 -> [w373] mode=indexing
              tunnel: [w374] -> w346 mode=indexing
              n214 = Build Array(0.0 ("element"), w373, w372) -> (w374:dbl[])
            }
            n215 = call "UpdateSpotMap.vi"("Rawdata"=w345, "Coefficients"=w346, "Mask (input)"=w344, "Display Input"=w343, "radius"="radius", "error in (no error)"=w365) -> ("Mask (output)"=w361:T1, "Display (output"=w360:T1, "error out"=w367:errorcluster)
            n216 = Bundle By Name(cluster=w370, "Mask"=w361, "Display"=w360, "Coefficients (2D)"=w346) -> (w368:T7)
            n217 = call "HandleError.vi"("error in (no error)"=w367) -> ()
            n218 = call "PickImage.vi"("Get/Set"=TRUE, "Images (input)"=w368) -> ()  [unwired: 1 out]
          }
          event #4 {
            n219 = event-data() -> ()  [unwired: 1 in, 5 out]
            n220 = call "PickImage.vi"() -> ("Image (output)"=w388:T7)  [unwired: 2 in]
            n221 = Unbundle By Name(w388) -> ("Rawdata"=w383:T1, "Mask"=w382:T1, "Display"=w381:T1, "Coefficients (2D)"=w384:sgl[][])
            n222 = local read "Pick Settings"() -> (w377:T3)
            n223 = Unbundle By Name(w377) -> ("radius"=w376:i32)
            n224 = call "UpdateSpotMap.vi"("Rawdata"=w383, "Coefficients"=w384, "Mask (input)"=w382, "Display Input"=w381, "radius"=w376) -> ("Mask (output)"=w380:T1, "Display (output"=w379:T1, "error out"=w378:errorcluster)  [unwired: 1 in]
            n225 = call "HandleError.vi"("error in (no error)"=w378) -> ()
            n226 = call "PickImage.vi"() -> ("Image (output)"=w387:T7)  [unwired: 2 in]
            n227 = Bundle By Name(cluster=w387, "Mask"=w380, "Display"=w379) -> (w385:T7)
            n228 = call "PickImage.vi"("Get/Set"=TRUE, "Images (input)"=w385) -> ()  [unwired: 1 out]
          }
          event #5 {
            n229 = event-data() -> ()  [unwired: 1 in, 5 out]
            n230 = stacked-sequence {
              frame #0 {
                w389 = u16 1 items=["standalone", "dialog"] ("mode")
                n231 = call "DAQFIFO_HH.vi"("mode"=w389) -> ()
              }
              frame #1 {
                n232 = call "FIFOSettings.vi"() -> ("FIFO Settings(out)"=w390:T6)  [unwired: 2 in]
                n233 = Unbundle By Name(w390) -> ("Measurement.Binning (ms)"=w394:sgl)
                n234 = call "SPCSetParameters_HH.vi"("FIFO Settings"=w390) -> ("error (out)"=w395:errorcluster)  [unwired: 2 in]
                n235 = call "HandleError.vi"("error in (no error)"=w395) -> ()
                n236 = Reciprocal(x=w394) -> (1/x=w393:sgl)
                n237 = Multiply(x=w393, y=sgl 1000.0) -> (x*y=w392:sgl)
                n238 = property on="MCS" class="WFChart (strict)"("X Scale.Offset and Multiplier:Multiplier"=w392) -> ()  [unwired: 2 in, 2 out]
              }
            }
          }
          event #6 {
            n239 = event-data() -> ()  [unwired: 1 in, 5 out]
            n240 = call "SetupEOM.vi"() -> ()  [unwired: 1 in]
          }
          event #7 {
            n241 = event-data() -> ()  [unwired: 1 in, 6 out]
            n242 = call "SetupAOTF.vi"() -> ()  [unwired: 1 in]
          }
          event #8 {
            n243 = event-data() -> ()  [unwired: 1 in, 5 out]
            n244 = case shown="True" "Stage Setup" {
              frame #0 {
              }
              frame #1 {
                n245 = stacked-sequence {
                  seq-local: [w397 _ _] -> [_ _ w399]
                  frame #0 {
                    n246 = call "StageType.vi"() -> ("Stage Type (output)"=w397:T11)  [unwired: 3 in, 2 out]
                  }
                  frame #1 {
                    n247 = call "SetupStage.vi"() -> ()  [unwired: 1 in]
                  }
                  frame #2 {
                    n248 = call "StageType.vi"() -> ("Stage Type (output)"=w400:T11)  [unwired: 3 in, 2 out]
                    n249 = Not Equal?(x=w399, y=w400) -> (x != y?=w398:bool)
                    n250 = case shown="True" w398 {
                      frame #0 {
                      }
                      frame #1 {
                        n251 = call "StageInit.vi"() -> ("error out"=w401:errorcluster)  [unwired: 1 in]
                        n252 = call "HandleError.vi"("error in (no error)"=w401) -> ()
                      }
                    }
                  }
                }
              }
            }
          }
          event #9 {
            n253 = event-data() -> ()  [unwired: 1 in, 6 out]
            n254 = flat-sequence {
              frame #0 {
                n255 = call "RampSetup.vi"() -> ()  [unwired: 1 in]
              }
              frame #1 {
                n256 = call "RampSetting.vi"() -> ("RampSetting (out)"=w403:T12)  [unwired: 2 in]
                n257 = Unbundle By Name(w403) -> ("used"=→"used":bool)
              }
            }
          }
          event #10 {
            n258 = event-data() -> ()  [unwired: 1 in, 5 out]
            n259 = call "PickImage.vi"() -> ("Image (output)"=w405:T7)  [unwired: 2 in]
            n260 = Unbundle By Name(w405) -> ("Display"=w404:T1)
            n261 = call "SaveIMAQImage.vi"("IMAQ Image"=w404) -> ()
          }
          event #11 {
            n262 = event-data() -> ()  [unwired: 1 in, 5 out]
            n263 = case shown="True" "Run" {
              frame #0 {
                w408 = FALSE ("Laser 1")
                n264 = property on=".sm file format" class="Bool (strict)"() -> ("Value"=w407:bool)  [unwired: 2 in, 2 out]
                n265 = call "FIFOStopDAQ.vi"() -> ("error out"=w411:errorcluster)
                n266 = call "OperateOnAnalogOutput.vi"("error in (no error)"=w411, "operation"=enum16{"start", "state", "abort"}."abort") -> ("error out"=w410:errorcluster)  [unwired: 1 out]
                n267 = call "FIFOFileObject.vi"(".sm file format"=w407, "function (open:0)"=enum16{"open", "write", "close"}."close", "error in (no error)"=w410) -> ("error out"=w412:errorcluster)  [unwired: 3 in]
                n268 = call "AOTFSetPosition.vi"() -> ()  [unwired: 2 in]
                n269 = call "HandleError.vi"("error in (no error)"=w412) -> ()
                n270 = property on="Laser 2" class="Boolean (strict)"("Value"=w408) -> ()  [unwired: 2 in, 2 out]
                n271 = property on="Laser 3" class="Boolean (strict)"("Value"=w408) -> ()  [unwired: 2 in, 2 out]
                n272 = property on="Laser 1" class="Boolean (strict)"("Value"=w408) -> ()  [unwired: 2 in, 2 out]
                n273 = property on="Laser 4" class="Boolesch (strikt)"("Value"=w408) -> ()  [unwired: 2 in, 2 out]
              }
              frame #1 {
                n274 = stacked-sequence {
                  frame #0 {
                    n275 = flat-sequence {
                      frame #0 {
                        n276 = call "RampSetting.vi"() -> ("RampSetting (out)"=w415:T12)  [unwired: 2 in]
                        n277 = Unbundle By Name(w415) -> ("used"=w414:bool)
                        n278 = case shown="False" w414 {
                          tunnel: "AOTF" -> [w417 w421]
                          frame #0 {
                            n279 = call "InitializeAnalogOutputforPAD.vi"("AOTF"=w417, "% puls-duration"="% puls-duration", "% rel. duration"="% duration Laser1", "EOM"="EOM") -> ()
                          }
                          frame #1 {
                            n280 = call "InitializeAnalogOutputforPADwithRamp.vi"("AOTF"=w421) -> ()  [unwired: 3 in]
                          }
                        }
                      }
                      frame #1 {
                        w423 = u16 0 items=["init", "run"] ("mode")
                        w424 = u32 0 ("Destroy Index")
                        n281 = property on="Actual Spot No." class="Digital (strict)"("Value"=w424) -> ()  [unwired: 2 in, 2 out]
                        n282 = call "FIFOInitDAQ_HH.vi"() -> ()  [unwired: 1 in]
                        n283 = call "PickImage.vi"() -> ("Image (output)"=w427:T7)  [unwired: 2 in]
                        n284 = Bundle By Name(cluster=w427, "Destroy Index"=w424) -> (w426:T7)
                        n285 = call "PickImage.vi"("Get/Set"=TRUE, "Images (input)"=w426) -> ()  [unwired: 1 out]
                        n286 = call "_updateOnlineDisplay_LV.vi"("show lifetime"=FALSE, "mode"=w423) -> ()  [unwired: 2 in, 2 out]
                      }
                    }
                  }
                  frame #1 {
                    n287 = call "TestDestroyIndex.vi"() -> ("Boolean"=w428:bool, "Destroy Index"=w429:u32)
                    n288 = case shown="True" w428 {
                      tunnel: w429 -> [_ w431]
                      frame #0 {
                        n289 = property on="Run" class="Boolean (strict)"("Value"=FALSE ("Run")) -> ()  [unwired: 2 in, 2 out]
                      }
                      frame #1 {
                        n290 = stacked-sequence {
                          seq-local: [_ w435 _ _] -> [_ _ _ w463]
                          tunnel: w431 -> [w432 w433 _ _]
                          frame #0 {
                            n291 = property on="Actual Spot No." class="DigNum (strict)"("Value"=w432) -> ()  [unwired: 2 in, 2 out]
                          }
                          frame #1 {
                            n292 = property on="Store Data" class="Bool (strict)"() -> ("Value"=w434:bool)  [unwired: 2 in, 2 out]
                            n293 = case shown="True" w434 {
                              tunnel: [_ w443] -> w435
                              tunnel: w433 -> [_ w438]
                              frame #0 {
                              }
                              frame #1 {
                                n294 = property on="Destination:" class="Path"() -> ("Value"=w439:path)  [unwired: 2 in, 2 out]
                                n295 = Format Into String(format string="spot%03d.fifo", w438) -> (resulting string=w441:string, error out=w440:errorcluster)  [unwired: 2 in]
                                n296 = Build Path(base path=w439, name or relative path=w441) -> (appended path=w437:path)
                                n297 = call "WriteFIFOHeader_HH.vi"("error in"=w440, "Destination:"=w437) -> ("error out"=w444:errorcluster)
                                n298 = call "FIFOFileObject.vi"(".sm file format"=".sm file format", "function (open:0)"=enum16{"open", "write", "close"}."open", "error in (no error)"=w444, "Destination:"=w437) -> ("error out"=w443:errorcluster)  [unwired: 2 in]
                              }
                            }
                          }
                          frame #2 {
                            w452 = u16 0 items=["initialize", "test limit"] ("operation")
                            n299 = property on="Image Settings" class="Clust (strict)"() -> ("Value"=w448:T10)  [unwired: 2 in, 2 out]
                            n300 = call "FIFOSettings.vi"() -> ("FIFO Settings(out)"=w453:T6)  [unwired: 2 in]
                            n301 = Unbundle By Name(w453) -> ("Measurement"=w451:T8, "Measurement.Stop Condition:"=w454:u16)
                            n302 = call "UpdateDestroyPosition.vi"("AFM Mode"="AFM mode", "Image Settings"=w448) -> ("error out"=w447:errorcluster)  [unwired: 1 in]
                            n303 = property on="MCS" class="WFChart (strict)"("History Data"=u32[][] []) -> ()  [unwired: 2 in, 2 out]
                            n304 = call "HandleError.vi"("error in (no error)"=w447) -> ()
                            n305 = case shown="0, Default" w454 {
                              tunnel: [_ u32 0 ("Start (input)") w457] -> w449
                              frame #0 {
                              }
                              frame #1 {
                              }
                              frame #2 {
                                n306 = Tick Count (ms)() -> (millisecond timer value=w457:u32)
                              }
                            }
                            n307 = call "FIFOStart.vi"("Set/Get"=TRUE, "Start (input)"=w449) -> ()  [unwired: 1 out]
                            n308 = call "IsFIFOFinished_HH.vi"("Measurement"=w451, "Time"=w449, "Counts"=w449, "operation"=w452) -> ()  [unwired: 1 out]
                          }
                          frame #3 {
                            n309 = call "StageType.vi"("Function"=T5."Get Type") -> ("Stage Type (output)"=w458:T11)  [unwired: 2 in, 2 out]
                            n310 = case shown="No Error" w463 {
                              selector: w463 -> [_ w469]
                              tunnel: [w465 w469] -> w460
                              tunnel: w458 -> [w464 _]
                              frame #0 {
                                n311 = case shown="\"PI 725 USB\", \"PI 725 TCP/IP\"" w464 {
                                tunnel: [w466 w468] -> w465
                                frame #0 {
                                w467 = u16 0 items=["start", "state", "abort"] ("operation")
                                n312 = call "OperateOnAnalogOutput.vi"("operation"=w467) -> ("error out"=w466:errorcluster)  [unwired: 1 in, 1 out]
                                }
                                frame #1 {
                                n313 = call "FIFOStartDAQ_HH.vi"() -> ("error out"=w468:errorcluster)  [unwired: 1 in]
                                }
                                }
                              }
                              frame #1 {
                              }
                            }
                            n314 = Unbundle By Name(w460) -> ("status"=w462:bool)
                            n315 = call "HandleError.vi"("error in (no error)"=w460) -> ()
                            n316 = Not(x=w462) -> (.not. x?=w461:bool)
                            n317 = property on="Run" class="Bool (strict)"("Value"=w461) -> ()  [unwired: 2 in, 2 out]
                          }
                        }
                      }
                    }
                  }
                  frame #2 {
                    n318 = property on="Store Data" class="Boolesch (strikt)"() -> ("Value"=w470:bool)  [unwired: 2 in, 2 out]
                    n319 = case shown="False" w470 {
                      frame #0 {
                      }
                      frame #1 {
                        n320 = call "DAQLinescanVisualization.vi"() -> ("Visualization (output)"=w476:T13)  [unwired: 2 in]
                        n321 = property on="Destination:" class="Pfad"() -> ("Value"=w473:path)  [unwired: 2 in, 2 out]
                        n322 = Unbundle By Name(w476) -> ("IMAQ Trace"=w475:T1)
                        n323 = Build Path(base path=w473, name or relative path="SpotMap.png" ("Name oder relativer Pfad")) -> (appended path=w474:path)
                        n324 = call "IMAQ WriteFile"("File Type"="png", "File Path"=w474, "Image"=w475) -> ()  [unwired: 5 in, 1 out]
                      }
                    }
                  }
                }
              }
            }
          }
          event #12 {
            n325 = event-data() -> ("NewVal"=w478:u16)  [unwired: 1 in, 5 out]
            n326 = Not Equal To 0?(x=w478) -> (x != 0?=w477:bool)
            n327 = case shown="True" w477 {
              frame #0 {
                w479 = u8 0 ("Disabled")
                n328 = property on="Laser 1" class="Boolean (strict)"("Disabled"=w479) -> ()  [unwired: 2 in, 2 out]
                n329 = property on="Laser 2" class="Bool (strict)"("Disabled"=w479) -> ()  [unwired: 2 in, 2 out]
                n330 = property on="Laser 3" class="Bool (strict)"("Disabled"=w479) -> ()  [unwired: 2 in, 2 out]
                n331 = property on="Laser 4" class="Boolesch (strikt)"("Disabled"=w479) -> ()  [unwired: 2 in, 2 out]
              }
              frame #1 {
                w481 = FALSE ("Laser 1")
                w480 = u8 2 ("Disabled")
                n332 = call "AOTFSetPosition.vi"() -> ()  [unwired: 2 in]
                n333 = property on="Laser 1" class="Boolean (strict)"("Disabled"=w480, "Value"=w481) -> ()  [unwired: 2 in, 2 out]
                n334 = property on="Laser 2" class="Boolean (strict)"("Disabled"=w480, "Value"=w481) -> ()  [unwired: 2 in, 2 out]
                n335 = property on="Laser 3" class="Boolean (strict)"("Disabled"=w480, "Value"=w481) -> ()  [unwired: 2 in, 2 out]
                n336 = property on="Laser 4" class="Boolesch (strikt)"("Disabled"=w480, "Value"=w481) -> ()  [unwired: 2 in, 2 out]
              }
            }
          }
          event #13 {
            n337 = event-data() -> ()  [unwired: 1 in, 6 out]
            n338 = call "AOTFSettings.vi"() -> ("AOTF Setting (Output)"=w486:T14)  [unwired: 2 in]
            n339 = call "AnalogSettings.vi"() -> ("Analog Settings (output)"=w487:T15)  [unwired: 2 in]
            n340 = Unbundle By Name(w487) -> ("PCI 671x Device Number"=w485:u32)
            n341 = Unbundle By Name(w486) -> ("Laser 1 Output Channel"=w484:tag, "AOTF  1 Output Voltage"=w483:dbl)
            n342 = case shown="False" "Laser 1" {
              tunnel: w485 -> [w488 w493]
              tunnel: w484 -> [w489 w492]
              tunnel: w483 -> [_ w491]
              frame #0 {
                n343 = call-poly "AO Update Channel.vi"("value"=sgl 0.0, "channel (0)"=w489, "device"=w488) -> ()
              }
              frame #1 {
                n344 = call-poly "AO Update Channel.vi"("value"=w491, "channel (0)"=w492, "device"=w493) -> ()
              }
            }
          }
          event #14 {
            n345 = event-data() -> ()  [unwired: 1 in, 6 out]
            n346 = call "AOTFSettings.vi"() -> ("AOTF Setting (Output)"=w498:T14)  [unwired: 2 in]
            n347 = call "AnalogSettings.vi"() -> ("Analog Settings (output)"=w499:T15)  [unwired: 2 in]
            n348 = Unbundle By Name(w499) -> ("PCI 671x Device Number"=w497:u32)
            n349 = Unbundle By Name(w498) -> ("Laser 2 Output Channel"=w496:tag, "AOTF  2 Output Voltage"=w495:dbl)
            n350 = case shown="False" "Laser 2" {
              tunnel: w497 -> [w500 w505]
              tunnel: w496 -> [w501 w504]
              tunnel: w495 -> [_ w503]
              frame #0 {
                n351 = call-poly "AO Update Channel.vi"("value"=sgl 0.0, "channel (0)"=w501, "device"=w500) -> ()
              }
              frame #1 {
                n352 = call-poly "AO Update Channel.vi"("value"=w503, "channel (0)"=w504, "device"=w505) -> ()
              }
            }
          }
          event #15 {
            n353 = event-data() -> ()  [unwired: 1 in, 6 out]
            n354 = call "AOTFSettings.vi"() -> ("AOTF Setting (Output)"=w509:T14)  [unwired: 2 in]
            n355 = call "AnalogSettings.vi"() -> ("Analog Settings (output)"=w510:T15)  [unwired: 2 in]
            n356 = Unbundle By Name(w510) -> ("PCI 671x Device Number"=w508:u32)
            n357 = Unbundle By Name(w509) -> ("Laser 3 Output Channel"=w507:tag, "AOTF  3 Output Voltage"=w506:dbl)
            n358 = case shown="False" "Laser 3" {
              tunnel: w508 -> [w512 w517]
              tunnel: w507 -> [w513 w516]
              tunnel: w506 -> [_ w515]
              frame #0 {
                n359 = call-poly "AO Update Channel.vi"("value"=sgl 0.0, "channel (0)"=w513, "device"=w512) -> ()
              }
              frame #1 {
                n360 = call-poly "AO Update Channel.vi"("value"=w515, "channel (0)"=w516, "device"=w517) -> ()
              }
            }
          }
          event #16 {
            n361 = event-data() -> ()  [unwired: 1 in, 6 out]
            n362 = call "AOTFSettings.vi"() -> ("AOTF Setting (Output)"=w522:T14)  [unwired: 2 in]
            n363 = call "AnalogSettings.vi"() -> ("Analog Settings (output)"=w523:T15)  [unwired: 2 in]
            n364 = Unbundle By Name(w523) -> ("PCI 671x Device Number"=w521:u32)
            n365 = Unbundle By Name(w522) -> ("Laser 4 Output Channel"=w520:tag, "AOTF  4 Output Voltage"=w519:dbl)
            n366 = case shown="True" "Laser 4" {
              tunnel: w521 -> [w524 w529]
              tunnel: w520 -> [w525 w528]
              tunnel: w519 -> [_ w527]
              frame #0 {
                n367 = call-poly "AO Update Channel.vi"("value"=sgl 0.0, "channel (0)"=w525, "device"=w524) -> ()
              }
              frame #1 {
                n368 = call-poly "AO Update Channel.vi"("value"=w527, "channel (0)"=w528, "device"=w529) -> ()
              }
            }
          }
          event #17 {
            n369 = event-data() -> ()  [unwired: 1 in, 5 out]
            n370 = stacked-sequence {
              frame #0 {
                n371 = call "offset.vi"("set?"=TRUE, "offset"="offset (pixel)") -> ()  [unwired: 1 in, 1 out]
              }
              frame #1 {
                n372 = property on="Image Settings" class="Clust (strict)"() -> ("Value"=w532:T10)  [unwired: 2 in, 2 out]
                n373 = call "UpdateDestroyPositionJustOffset.vi"("Image Settings"=w532) -> ("error out"=w533:errorcluster)  [unwired: 1 in]
                n374 = call "HandleError.vi"("error in (no error)"=w533) -> ()
              }
            }
          }
          event #18 {
            w534 = TRUE
            n375 = event-data() -> ()  [unwired: 1 in, 5 out]
            n376 = call "PickImage.vi"() -> ("Image (output)"=w538:T7)  [unwired: 2 in]
            n377 = Unbundle By Name(w538) -> ("Rawdata"=w537:T1, "Mask"=w536:T1, "Display"=w535:T1)
            n378 = call "IMAQ Dispose"("Image"=w537) -> ()  [unwired: 5 in, 1 out]
            n379 = call "IMAQ Dispose"("Image"=w536) -> ()  [unwired: 5 in, 1 out]
            n380 = call "IMAQ Dispose"("Image"=w535) -> ()  [unwired: 5 in, 1 out]
            "Boolean" <- w534
          }
        }
      }
      n381 = while {
        stop <- w61 stop-if-true
        n382 = event shown="[0] \"Automate Mesaurement \": Value Change" {
          selector: _ -> [_ _]
          dyn-events: _ -> [_ _]
          timeout: _ -> [_ _]
          event #0 {
            n383 = event-data() -> ()  [unwired: 1 in, 5 out]
            n384 = local read "NrOfSpots"() -> (w64:i32)
            n385 = for {
              N: w64 -> [_]
              tunnel: w64 -> [w66]
              tunnel: [w65] -> w63
              n386 = property on="Run" class="Bool (strict)"() -> ("Value"=w69:bool)  [unwired: 2 in, 2 out]
              n387 = Greater?(x=w66, y=0) -> (0:w68:bool)
              n388 = Not(x=w69) -> (.not. x?=w70:bool)
              n389 = And(x=w70, y=w68) -> (x .and. y?=w67:bool)
              n390 = case shown="True" w67 {
                tunnel: [_ w140] -> w73
                frame #0 {
                }
                frame #1 {
                  n391 = property on="Automate Mesaurement" class="Bool (strict)"() -> (error out=w142:errorcluster, "Value"=w141:bool)  [unwired: 2 in, 1 out]
                  n392 = case shown="False" w141 {
                    tunnel: [w143 w144] -> w140
                    tunnel: w142 -> [w143 w144]
                    frame #0 {
                    }
                    frame #1 {
                      n393 = Wait (ms)(milliseconds to wait=u32 500) -> ()  [unwired: 1 out]
                    }
                  }
                }
              }
              n394 = case shown="True" "AutoFocus Z" {
                tunnel: w73 -> [w135 w139]
                tunnel: [w135 w138] -> w71
                frame #0 {
                }
                frame #1 {
                  n395 = property on="autofocus stub" class="Arr (strict)"(error in=w139) -> (error out=w138:errorcluster, "Value"=w137:i32[])  [unwired: 1 in, 1 out]
                  n396 = Add Array Elements(numeric array=w137) -> (sum=→"sum":i32)
                }
              }
              n397 = stacked-sequence {
                tunnel: w71 -> [_ _ _]
                tunnel: [_ _ w133] -> w65
                frame #0 {
                  n398 = call "PickImage.vi"() -> ("Image (output)"=w78:T7)  [unwired: 2 in]
                  n399 = Unbundle By Name(w78) -> ("Destroy Index"=w76:u32)
                  n400 = stacked-sequence {
                    frame #0 {
                      n401 = call "FIFOStopDAQ.vi"() -> ("error out"=w80:errorcluster)
                      n402 = call "HandleError.vi"("error in (no error)"=w80) -> ()
                    }
                    frame #1 {
                      w82 = u16 2 items=["start", "state", "abort"] ("operation")
                      n403 = call "OperateOnAnalogOutput.vi"("operation"=w82) -> ("error out"=w81:errorcluster)  [unwired: 1 in, 1 out]
                      n404 = call "HandleError.vi"("error in (no error)"=w81) -> ()
                    }
                    frame #2 {
                      n405 = property on=".sm file format" class="Bool (strict)"() -> ("Value"=w83:bool)  [unwired: 2 in, 2 out]
                      n406 = call "FIFOFileObject.vi"(".sm file format"=w83, "function (open:0)"=enum16{"open", "write", "close"}."close") -> ()  [unwired: 4 in, 1 out]
                    }
                    frame #3 {
                      n407 = property on="EOM" class="Ring (strict)"() -> ("Value"=w86:u16)  [unwired: 2 in, 2 out]
                      n408 = property on="AOTF" class="Ring (strict)"() -> ("Value"=w85:u16)  [unwired: 2 in, 2 out]
                      n409 = Equal To 0?(x=w86) -> (x = 0?=w88:bool)
                      n410 = Equal To 0?(x=w85) -> (x = 0?=w87:bool)
                      n411 = case shown="True" w88 {
                        frame #0 {
                          n412 = call "EOMSetPosition.vi"("value"=sgl 0.0) -> ()
                        }
                        frame #1 {
                        }
                      }
                      n413 = case shown="False" w87 {
                        frame #0 {
                          n414 = call "AOTFSetPosition.vi"() -> ()  [unwired: 2 in]
                        }
                        frame #1 {
                        }
                      }
                    }
                  }
                  n415 = Increment(x=w76) -> (x+1=w77:u32)
                  n416 = Bundle By Name(cluster=w78, "Destroy Index"=w77) -> (w79:T7)
                  n417 = call "PickImage.vi"("Get/Set"=TRUE, "Images (input)"=w79) -> ()  [unwired: 1 out]
                }
                frame #1 {
                  n418 = call "TestDestroyIndex.vi"() -> ("Boolean"=w91:bool, "Destroy Index"=w90:u32)
                  n419 = case shown="False" w91 {
                    tunnel: w90 -> [_ w94]
                    frame #0 {
                      w92 = FALSE ("Laser 1")
                      n420 = call "AOTFSetPosition.vi"() -> ()  [unwired: 2 in]
                      n421 = property on="Run" class="Bool (strict)"("Value"=FALSE ("Run")) -> ()  [unwired: 2 in, 2 out]
                      n422 = property on="Laser 4" class="Bool (strict)"("Value"=w92) -> ()  [unwired: 2 in, 2 out]
                      n423 = property on="Laser 1" class="Bool (strict)"("Value"=w92) -> ()  [unwired: 2 in, 2 out]
                      n424 = property on="Laser 3" class="Bool (strict)"("Value"=w92) -> ()  [unwired: 2 in, 2 out]
                      n425 = property on="Laser 2" class="Bool (strict)"("Value"=w92) -> ()  [unwired: 2 in, 2 out]
                    }
                    frame #1 {
                      n426 = stacked-sequence {
                        seq-local: [_ w98 _ _] -> [_ _ _ w126]
                        tunnel: w94 -> [w95 w97 _ _]
                        frame #0 {
                          n427 = property on="Actual Spot No." class="DigNum (strict)"("Value"=w95) -> ()  [unwired: 2 in, 2 out]
                        }
                        frame #1 {
                          n428 = property on="Store Data" class="Bool (strict)"() -> ("Value"=w96:bool)  [unwired: 2 in, 2 out]
                          n429 = case shown="True" w96 {
                            tunnel: [_ w107] -> w98
                            tunnel: w97 -> [_ w104]
                            frame #0 {
                            }
                            frame #1 {
                              n430 = Format Into String(format string="spot%03d.fifo", w104) -> (resulting string=w105:string, error out=w102:errorcluster)  [unwired: 2 in]
                              n431 = property on="Destination:" class="Path"() -> ("Value"=w101:path)  [unwired: 2 in, 2 out]
                              n432 = Build Path(base path=w101, name or relative path=w105) -> (appended path=w103:path)
                              n433 = call "WriteFIFOHeader_HH.vi"("error in"=w102, "Destination:"=w103) -> ("error out"=w100:errorcluster)
                              n434 = property on=".sm file format" class="Bool (strict)"() -> ("Value"=w99:bool)  [unwired: 2 in, 2 out]
                              n435 = call "FIFOFileObject.vi"(".sm file format"=w99, "function (open:0)"=enum16{"open", "write", "close"}."open", "error in (no error)"=w100, "Destination:"=w103) -> ("error out"=w107:errorcluster)  [unwired: 2 in]
                            }
                          }
                        }
                        frame #2 {
                          w115 = u16 0 items=["initialize", "test limit"] ("operation")
                          n436 = local read "AFM mode"() -> (w111:bool)
                          n437 = call "FIFOSettings.vi"() -> ("FIFO Settings(out)"=w116:T6)  [unwired: 2 in]
                          n438 = Unbundle By Name(w116) -> ("Measurement"=w114:T8, "Measurement.Stop Condition:"=w117:u16)
                          n439 = property on="Image Settings" class="Clust (strict)"() -> ("Value"=w110:T10)  [unwired: 2 in, 2 out]
                          n440 = call "UpdateDestroyPosition.vi"("AFM Mode"=w111, "Image Settings"=w110) -> ("error out"=w112:errorcluster)  [unwired: 1 in]
                          n441 = property on="MCS" class="WFChart (strict)"("Value"=u32[][] [] ("History Data")) -> ()  [unwired: 2 in, 2 out]
                          n442 = call "HandleError.vi"("error in (no error)"=w112) -> ()
                          n443 = case shown="2" w117 {
                            tunnel: [_ u32 0 ("Start (input)") w120] -> w113
                            frame #0 {
                            }
                            frame #1 {
                            }
                            frame #2 {
                              n444 = Tick Count (ms)() -> (millisecond timer value=w120:u32)
                            }
                          }
                          n445 = call "FIFOStart.vi"("Set/Get"=TRUE, "Start (input)"=w113) -> ()  [unwired: 1 out]
                          n446 = call "IsFIFOFinished_HH.vi"("Measurement"=w114, "Time"=w113, "Counts"=w113, "operation"=w115) -> ()  [unwired: 1 out]
                        }
                        frame #3 {
                          n447 = call "StageType.vi"("Function"=T5."Get Type") -> ("Stage Type (output)"=w122:T11)  [unwired: 2 in, 2 out]
                          n448 = case shown="No Error" w126 {
                            selector: w126 -> [_ w132]
                            tunnel: [w128 w132] -> w124
                            tunnel: w122 -> [w127 _]
                            frame #0 {
                              n449 = case shown="\"PI 725 TCP/IP\", Default" w127 {
                                tunnel: [w129 w130] -> w128
                                frame #0 {
                                n450 = call "FIFOStartDAQ_HH.vi"() -> ("error out"=w129:errorcluster)  [unwired: 1 in]
                                }
                                frame #1 {
                                w131 = u16 0 items=["start", "state", "abort"] ("operation")
                                n451 = call "OperateOnAnalogOutput.vi"("operation"=w131) -> ("error out"=w130:errorcluster)  [unwired: 1 in, 1 out]
                                }
                              }
                            }
                            frame #1 {
                            }
                          }
                          n452 = Unbundle By Name(w124) -> ("status"=w125:bool)
                          n453 = call "HandleError.vi"("error in (no error)"=w124) -> ()
                          n454 = Not(x=w125) -> (.not. x?=w121:bool)
                          n455 = property on="Run" class="Bool (strict)"("Value"=w121) -> ()  [unwired: 2 in, 2 out]
                        }
                      }
                    }
                  }
                }
                frame #2 {
                  n456 = call "Time Delay"("Delay Time (s)"="Delay Time (s)") -> ("error out"=w133:errorcluster)  [unwired: 10 in]
                }
              }
              "spots left" <- w66
            }
            n457 = property on="Automate Mesaurement" class="Bool (strict)"(error in=w63, "Value"=FALSE ("Automate Mesaurement")) -> ()  [unwired: 1 in, 2 out]
          }
          event #1 {
            n458 = event-data() -> ()  [unwired: 1 in, 2 out]
          }
        }
        n459 = property on="Boolean" class="Bool (strict)"() -> ("Value"=w61:bool)  [unwired: 2 in, 2 out]
      }
    }
  }
